vi "Set Trigger Timer Count.vi"(8 "error in (no error)":errorcluster, 9 "Trigger Count (1)":i32=1 min=1, 10 "Timer (1)":i32=1 min=1 max=4 step=1 format="%#.6g", 11 "VISA resource name":refnum<visa-resource-name>) -> (0 "error out":errorcluster, 3 "VISA resource name out":refnum<visa-resource-name>)   [LabVIEW 2017, in "Keithley 2450.lvlib"]
doc: "This vi sets the number of events to generate each time the timer detects its trigger event or is enabled as a timer or alarm."
uses:
  Keithley 2450.lvlib
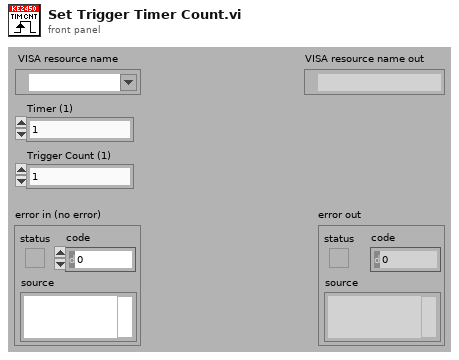
[diagram p1: front panel]
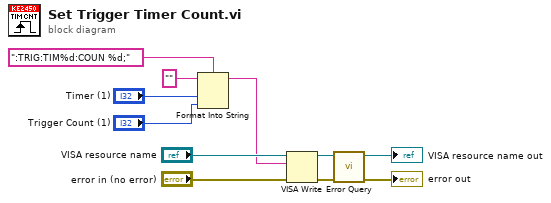
[diagram p0: block diagram]
diagram:
  n1 = Format Into String(format string=":TRIG:TIM%d:COUN %d;", initial string="", "Timer (1)", "Trigger Count (1)") -> (resulting string=w2:string)  [unwired: 1 in, 1 out]
  n2 = VISA Write(VISA resource name="VISA resource name", write buffer=w2, error in (no error)="error in (no error)") -> (VISA resource name out=w7:refnum<visa-resource-name>, error out=w6:errorcluster)  [unwired: 1 out]
  n3 = call "Error Query.vi"("error in (no error)"=w6, "VISA resource name"=w7) -> ("error out"=→"error out":errorcluster, "VISA resource name out"=→"VISA resource name out":refnum<visa-resource-name>)  [unwired: 8 out]
